vi "PH_Beamline.color Mirrortower BL.vi"(0 "i ref in":refnum<vi>, 2 "Color State MT Input":i32, 5 "error in (no error)":errorcluster) -> (14 "i ref out":refnum<vi>, 16 "Color State MT Exit Z6":i32, 19 "error out":errorcluster)   [LabVIEW 2014, in "PH_Beamline.lvlib"]
doc: "This Vi colors the Mirrortower beamline elements."
uses:
  PH_Beamline.lvlib
  PH_Basics/PH_StatusHandler/PH_StatusHandler.Status.ctl
  PH_Basics/PH_Common/PH_Common.lvlib
  PH_Basics/PH_StatusHandler/PH_StatusHandler.lvlib
  PH_BL-Master/PH_BL-Master.lvlib
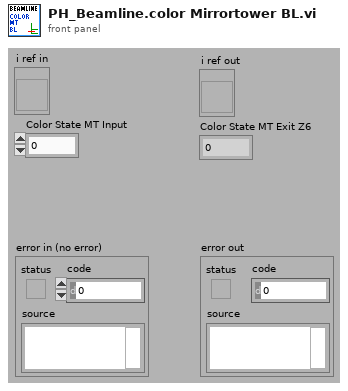
[diagram p1: front panel]
types:
  T1 = typedef "PH_StatusHandler.lvlib/PH_StatusHandler.Status.ctl" = i16
  T2 = typedef "PH_Beamline.lvlib/PH_Beamline.i attribute.ctl" = cluster{"GUI Refs":cluster{"PA ok":refnum<vi>, "MA ok":refnum<vi>, "fs FE ok":refnum<vi>, "ns FE ok":refnum<vi>, "PA ED ok":refnum<vi>, "MAS ok":refnum<vi>, "Booster ok":refnum<vi>, "Mirrortower ok":refnum<vi>, "In.-Box ok":refnum<vi>, "Compressor ok":refnum<vi>, "Experiment LB ok":refnum<vi>, "Experiment LL ok":refnum<vi>, "PHELIX_Beckhoff_Watchdog":refnum<vi>, "Shutters closed":refnum<vi>, "uOPA ok":refnum<vi>, "Vacuum no shotcond Comp LB":refnum<vi>}, "Refs BL MA":refnum<vi>[], "Refs BL MA-IB":refnum<vi>[], "Refs BL fs":refnum<vi>[], "Refs BL PA ED":refnum<vi>[], "Refs BL MAS":refnum<vi>[], "Refs BL Boo":refnum<vi>[], "Refs BL ns":refnum<vi>[], "Refs BL Mirrortower":refnum<vi>[], "Refs BL Compressor":refnum<vi>[], "Refs BL Exp LB":refnum<vi>[], "Radiation Safety":cluster{"Exp Laserbay":cluster{"Ref Op Mode":refnum<vi>, "Ref Laserbay evacuated":refnum<vi>, "Tagname LB evacuated":string, "Shot Mode":T3, "Laserbay evacuated?":i32, "Tagname HV room locked":string, "HV room locked?":i32, "Ref HV room locked":refnum<vi>, "Tagname bridged?":string, "Ref Bridge":refnum<vi>, "I<1E18W/cm²":bool}, "Exp Laserlab":cluster{"Ref Op Mode":refnum<vi>, "Ref Laserlab evacuated":refnum<vi>, "Tagname LL evacuated":string, "Shot Mode":T3, "Laserlab evacuated?":i32, "Tagname bridged?":string, "Ref Bridge":refnum<vi>, "I<1E18W/cm²":bool}}, "Refs BL LL":refnum<vi>[], "PP Igni Heating GUI Refs":refnum<vi>[], "PP Igni Heating Tagnames ":string[], "Refs BL PA":cluster{"undelayed Line before Shutter":refnum<vi>[], "undelayed Line after Shutter":refnum<vi>[], "before Bypass":refnum<vi>[], "delayed Line before Shutter":refnum<vi>[], "delayed Line after Shutter":refnum<vi>[], "before Shutter Input":refnum<vi>[], "after Shutter Input":refnum<vi>[], "Bypass":refnum<vi>[], "before Shutter Exit":refnum<vi>[], "after Shutter Exit":refnum<vi>[], "to MA":refnum<vi>[], "to Lab":refnum<vi>[]}, "BL":cluster{"YLF_BL_Status":i32, "fs_BL_Status":i32, "fs_YLF_BL_Status":i32, "ns_BL_Status":i32, "PA_Input_BL_Status":i32, "PA_UnDelay_BL_Status":i32, "PA_Delay_BL_Status":i32, "PA_BL_Status":i32, "PA_Bypass_BL_Status":i32, "PA_Exit_BL_Status":i32, "PA_LL_BL_Status":i32, "LL_BL_Status":i32, "PA_MA_BL_Status":i32, "MA_Exit_BL_Status":i32, "MA_Z6_BL_Status":i32, "Z6_BL_Status":i32, "MA_LB_BL_Status":i32, "LB_TB2_BL_Status":i32, "PA_before_Bypass_BL_Status":i32, "LB_TB3_BL_Status":i32}, "State Subsystems":cluster{"PA":bool, "MA":bool, "ns FE":bool, "fs FE":bool, "PA ED":bool, "In.-Box":bool, "MAS":bool, "Booster":bool, "Mirrortower":bool, "Compressor":bool, "Experiment LB":bool, "Experiment LL":bool, "uOPA":bool}, "Status Subscriber Information":T4, "Refs BL uOPA":refnum<vi>[], "PA_Input_2_Beam_6PWpGUI not linked?":bool, "PA_Input_Delay_6PGUI not linked?":bool, "Settings":T7}
  T3 = typedef "PH_Beamline.lvlib/PH_Beamline.Operation Mode.ctl" = i32
  T4 = typedef "PH_Beamline.lvlib/PH_Beamline.Status Subscriber Information.ctl" = cluster{"fs Swich YLF":T5, "fs Exit Shutter":T5, "ns Exit Shutter":T5, "PA Input Shutter":T5, "PA PC WP":T5, "PA PC WP 2":T5, "PA Bypass In":T5, "PA Bypass Out":T5, "PA CH 1":T5, "PA delayed":T5, "PA non delayed":T5, "PA Exit Shutter":T5, "PA Switch Lab":T5, "PA Bridge CH Input MA":T5, "MA Diffusor IB":T5, "MA IB Ready":T5, "MA CH 1":T5, "MA CH 2":T5, "MA CH 3":T5, "MA CH 4":T5, "MA Shutter Align Cam":T5, "MA Position MM5":T5, "Calorimeter Switch":T5, "BL Z6 CH 9":T5, "BL Z6 Beamdump":T5, "BL Z6 Shutter":T5, "COS Sensitivity Switch":T5, "Exp LB Shutter":T5, "Exp LB TB 2":T5, "Exp LB TB 3":T5, "PA LL Input CH":T5, "PA LL Output CH":T5, "LL Comp Input Shutter":T5, "LL Comp Output Shutter":T5, "LL Comp FF Shutter":T5, "Exp LL Shutter":T5, "MA IM In IB":T5, "MA IM Out IB":T5, "MA DB In IB":T5, "MA DB Out IB":T5, "Exp LB Shutter Interlock":T5, "Exp LL Shutter Interlock":T5, "MM1 Force Sensor":T5}
  T5 = typedef "PH_BL-Master.lvlib/PH_BL-Master.Status Subscriber Information.ctl" = cluster{"Index of element":i32, "Attributeset":T6}
  T6 = typedef "PH_BL-Master.lvlib/PH_BL-Master.Attribute Set.ctl" = enum16{"Boolean Status Service Subscriber", "Picture Status Service Subscriber"}
  T7 = typedef "PH_Beamline_Chief.lvlib/PH_Beamline_Chief.Settings.ctl" = cluster{"PA Doublepass Mode":bool, "Compressor Vaccuum LB not relevant":bool, "Windowshutter TB2 not relevant":bool, "Windowshutter TB3 not relevant":bool}
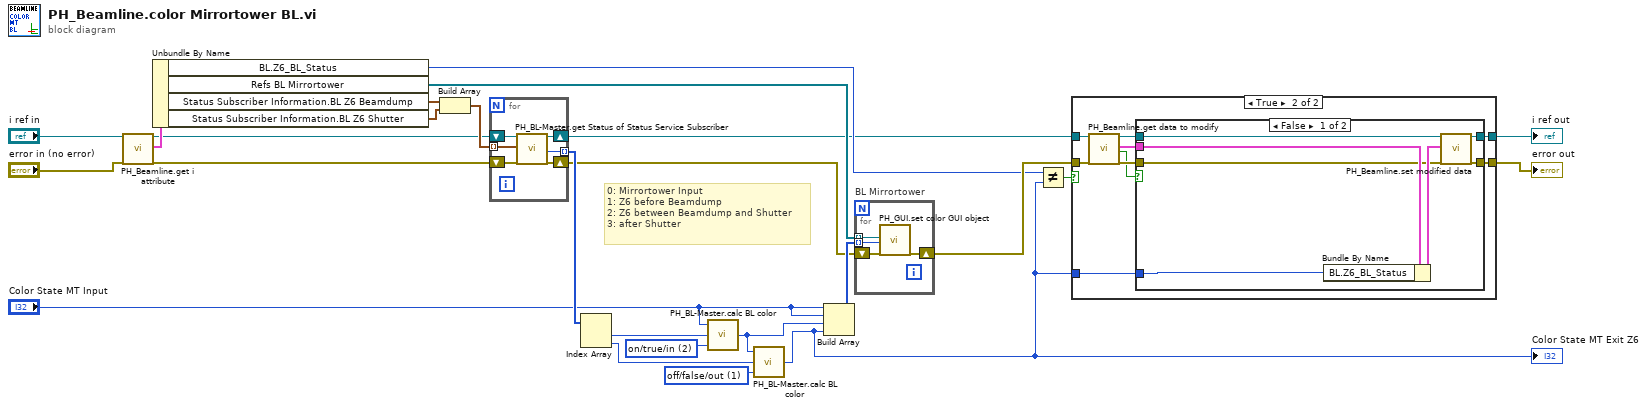
[diagram p0: block diagram]
diagram:
  w15 = T1 2 items=["no info", "off/false/out", "on/true/in", "Failure", "Alarm", "Status 1", "Status 2", "Status 3"] ("State for \"2\" (on) of ABLE (off/false/out)")
  w16 = T1 1 items=["no info", "off/false/out", "on/true/in", "Failure", "Alarm", "Status 1", "Status 2", "Status 3"] ("State for \"2\" (on) of ABLE (off/false/out)")
  # "0: Mirrortower Input\n1: Z6 before Beamdump\n2: Z6 between Beamdump and Shutter\n3: after Shutter"
  n1 = call "PH_Beamline.get i attribute.vi"("i ref in"="i ref in", "error in (no error)"="error in (no error)") -> ("i ref out"=w6:refnum<vi>, "i attribute"=w25:T2, "error out"=w5:errorcluster)  [unwired: 15 in]
  n2 = Unbundle By Name(w25) -> ("BL.Z6_BL_Status"=w11:i32, "Refs BL Mirrortower"=w24:refnum<vi>[], "Status Subscriber Information.BL Z6 Beamdump"=w2:T5, "Status Subscriber Information.BL Z6 Shutter"=w1:T5)
  n3 = Build Array(w2, w1) -> (w22:T5[])
  n4 = for {
    tunnel: [w31] -> w21 mode=indexing
    tunnel: w22 -> [w26] mode=indexing
    shift-right: [w27] -> w3
    shift-left: w5 -> [w28]
    shift-right: [w29] -> w4
    shift-left: w6 -> [w30]
    n5 = call "PH_BL-Master.get Status of Status Service Subscriber.vi"("i ref in"=w30, "Wanted Status Subscriber Information"=w26, "error in (no error)"=w28) -> ("i ref out"=w29:refnum<vi>, "Status"=w31:T1, "error out"=w27:errorcluster)  [unwired: 11 in, 3 out]
  }
  n6 = Index Array(array=w21) -> (element #1=w18:T1, element #2=w19:T1)  [unwired: 2 in]
  n7 = call "PH_BL-Master.calc BL color.vi"("State for \"2\" (on) of ABLE (off/false/out)"=w15, "State ABLE"=w18, "State before ABLE"="Color State MT Input") -> ("State after ABLE"=w20:i32)
  n8 = call "PH_BL-Master.calc BL color.vi"("State for \"2\" (on) of ABLE (off/false/out)"=w16, "State ABLE"=w19, "State before ABLE"=w20) -> ("State after ABLE"=w12:i32)
  "Color State MT Exit Z6" <- w12
  n9 = Build Array("Color State MT Input", "Color State MT Input", w20, w12) -> (w23:i32[])
  n10 = for "BL Mirrortower" {
    tunnel: w24 -> [w35] mode=indexing
    shift-right: [w33] -> w13
    shift-left: w3 -> [w34]
    tunnel: w23 -> [w32] mode=indexing
    n11 = call "PH_GUI.set color GUI object.vi"("GUI object Ref"=w35, "State"=w32, "error in (no error)"=w34) -> ("error out"=w33:errorcluster)  [unwired: 16 in]
  }
  n12 = Not Equal?(x=w11, y=w12) -> (x != y?=w14:bool)
  n13 = case shown="True" w14 {
    tunnel: w4 -> [w37 w42]
    tunnel: [w37 w41] -> w10
    tunnel: w13 -> [w36 w40]
    tunnel: [w36 w39] -> w9
    tunnel: w12 -> [_ w38]
    frame False {
    }
    frame True {
      n14 = call "PH_Beamline.get data to modify.vi"("i ref in"=w42, "error in (no error)"=w40) -> ("i ref out"=w45:refnum<vi>, "i attribute"=w43:T2, "timed out"=w44:bool, "error out"=w46:errorcluster)  [unwired: 14 in]
      n15 = case shown="False" w44 {
        tunnel: w46 -> [w47 w54]
        tunnel: w45 -> [w53 w55]
        tunnel: [w52 w54] -> w39
        tunnel: [w51 w55] -> w41
        tunnel: w43 -> [w48 _]
        tunnel: w38 -> [w49 _]
        frame False {
          n16 = Bundle By Name(cluster=w48, "BL.Z6_BL_Status"=w49) -> (w50:T2)
          n17 = call "PH_Beamline.set modified data.vi"("i ref in"=w53, "i attribute"=w50, "error in (no error)"=w47) -> ("i ref out"=w51:refnum<vi>, "error out"=w52:errorcluster)  [unwired: 15 in]
        }
        frame True {
        }
      }
    }
  }
  "error out" <- w9
  "i ref out" <- w10
